vi "pcb_query_command_tcp.vi"(8 "error in (no error)":errorcluster, 10 "command":string, 11 "connection ID":refnum<k5>) -> (0 "error out":errorcluster, 1 "bytes written":i32, 2 "output":string, 3 "connection ID out":refnum<k5>)   [LabVIEW 2018]
uses:
  <vilib>/Utility/error.llb/DialogType.ctl
panel:
  in  "Termination character":string=">>> "
  out "Numeric":i32
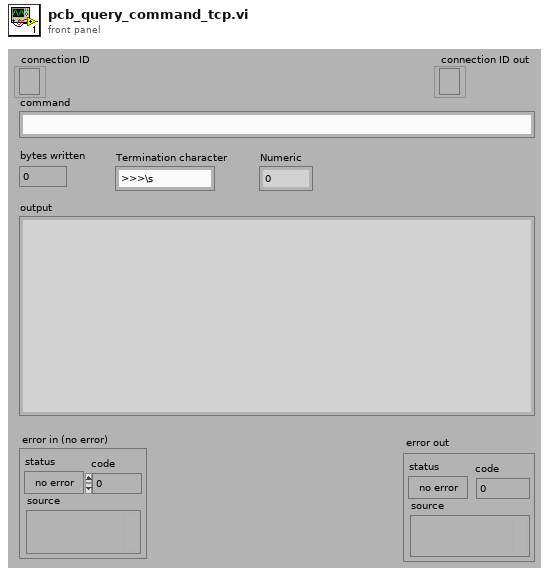
[diagram p1: front panel]
types:
  T1 = enum16{"Standard", "Buffered", "CRLF", "Immediate"}
  T2 = typedef "DialogType.ctl" = u16
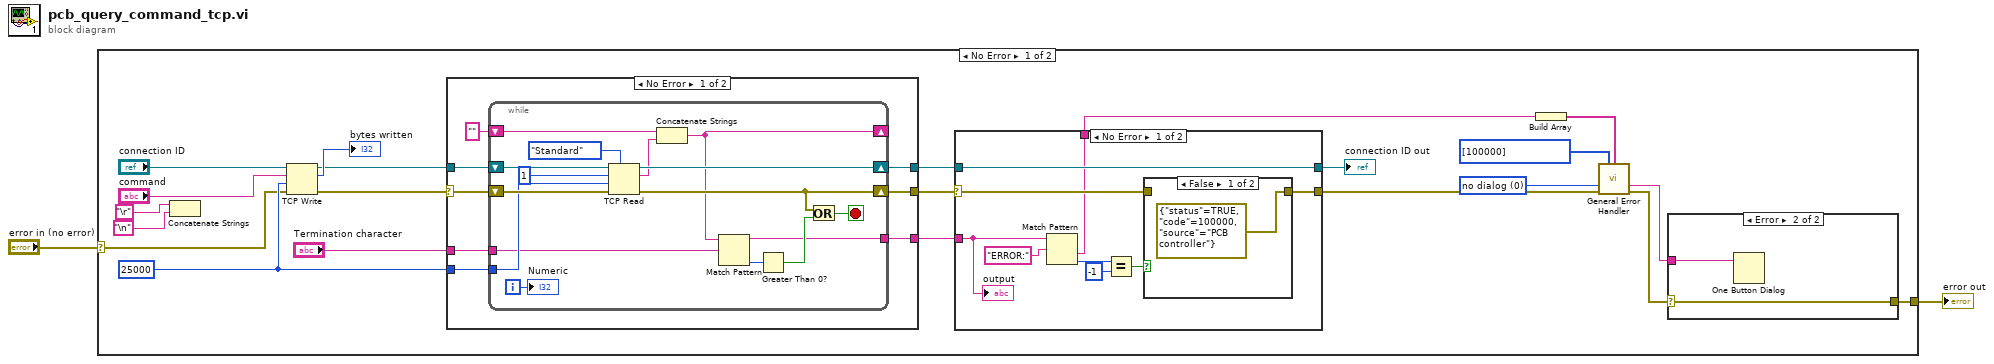
[diagram p0: block diagram]
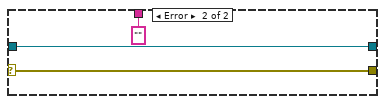
[diagram p4: hidden frame]
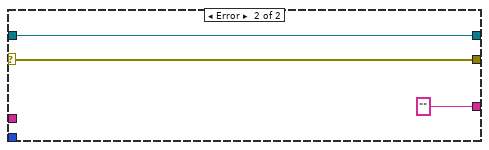
[diagram p5: hidden frame]
diagram:
  n1 = case shown="No Error" "error in (no error)" {
    selector: "error in (no error)" -> [w6 w69]
    tunnel: [w7 w69] -> w2
    frame No Error {
      w14 = 25000 ("timeout ms (25000)")
      w17 = T2 0 items=["no dialog", "OK message", "continue or stop message", "OK message + warnings", "continue/stop + warnings"] ("type of dialog (OK msg:1)")
      n2 = Concatenate Strings("\r", "\n") -> ()  [unwired: 1 out]
      n3 = TCP Write(connection ID="connection ID", data in="command", error in (no error)=w6, 9:w14) -> (connection ID out=w13:refnum<k5>, bytes written=→"bytes written":i32, error out=w12:errorcluster)
      n4 = case shown="No Error" w12 {
        selector: w12 -> [w47 w67]
        tunnel: [w49 w68] -> w21
        tunnel: w13 -> [w48 w68]
        tunnel: [w44 w67] -> w19
        tunnel: w14 -> [w46 _]
        tunnel: "Termination character" -> [w43 _]
        tunnel: [w42 "" ("data out")] -> w10
        frame No Error {
          n5 = while {
            shift-right: [w65] -> w49
            shift-left: w48 -> [w62]
            shift-right: [w55] -> w44
            shift-left: w47 -> [w59]
            shift-right: [w54] -> _
            shift-left: "" -> [w57]
            tunnel: w46 -> [w58]
            tunnel: w43 -> [w53]
            tunnel: [w50] -> w42
            i -> [w64]
            stop <- w56 stop-if-true
            n6 = TCP Read(connection ID=w62, bytes to read=1, error in (no error)=w59, 7:T1."Standard" ("mode (standard)"), 9:w58) -> (connection ID out=w65:refnum<k5>, data out=w63:string, error out=w55:errorcluster)
            n7 = Concatenate Strings(w57, w63) -> (w54:string)
            n8 = Match Pattern(string=w54, regular expression=w53) -> (before substring=w50:string, offset past match=w52:i32)  [unwired: 1 in, 2 out]
            n9 = Greater Than 0?(x=w52) -> (x > 0?=w51:bool)
            n10 = Or(x=w55, y=w51) -> (x .or. y?=w56:bool)
            "Numeric" <- w64
          }
        }
        frame Error {
        }
      }
      n11 = case shown="No Error" w19 {
        selector: w19 -> [w34 w41]
        tunnel: [w35 w41] -> w18
        tunnel: w21 -> [w33 w40]
        tunnel: [w33 w40] -> w20
        tunnel: w10 -> [w29 _]
        tunnel: [w28 "" ("data out")] -> w5
        frame No Error {
          n12 = Match Pattern(string=w29, regular expression="ERROR:" ("search string")) -> (after substring=w28:string, offset past match=w30:i32)  [unwired: 1 in, 2 out]
          n13 = Equal?(x=w30, y=-1) -> (x = y?=w32:bool)
          n14 = case shown="False" w32 {
            tunnel: w34 -> [_ w38]
            tunnel: [errorcluster {"status"=TRUE, "code"=100000, "source"="PCB controller"} ("error in (no error) 2") w38] -> w35
            frame False {
            }
            frame True {
            }
          }
          "output" <- w29
        }
        frame Error {
        }
      }
      "connection ID out" <- w20
      n15 = Build Array(w5) -> (w9:string[])
      n16 = call <vilib>:"General Error Handler.vi"("[user-defined codes]"=i32[] [100000], "[user-defined descriptions]"=w9, "type of dialog (OK msg:1)"=w17, "error in (no error)"=w18) -> ("message"=w15:string, "error out"=w8:errorcluster)  [unwired: 7 in, 3 out]
      n17 = case shown="Error" w8 {
        selector: w8 -> [w25 w26]
        tunnel: w15 -> [_ w27]
        tunnel: [w25 w26] -> w7
        frame No Error {
        }
        frame Error {
          n18 = One Button Dialog(message=w27) -> ()  [unwired: 1 in, 1 out]
        }
      }
    }
    frame Error {
    }
  }
  "error out" <- w2
